vi "Find Labelled Disable Structure.vi"(8 "error in (no error)":errorcluster, 10 "Label":string, 11 "VI in":refnum<vi>) -> (0 "error out":errorcluster, 1 "Found?":bool, 2 "DisableStructure Refnum":refnum<vi>)   [LabVIEW 2018]
uses:
  <vilib>/Utility/traverseref.llb/TRef TravTarget.ctl
  <vilib>/Utility/error.llb/Error Cluster From Error Code.vi
  <vilib>/ErrorRing/Error Ring.xnode
  <vilib>/Utility/traverseref.llb/VI Scripting - Traverse.lvlib
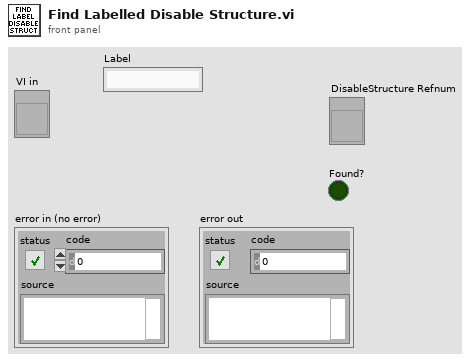
[diagram p1: front panel]
types:
  T1 = typedef "TRef TravTarget.ctl" = enum16{"FP", "BD", "Other"}
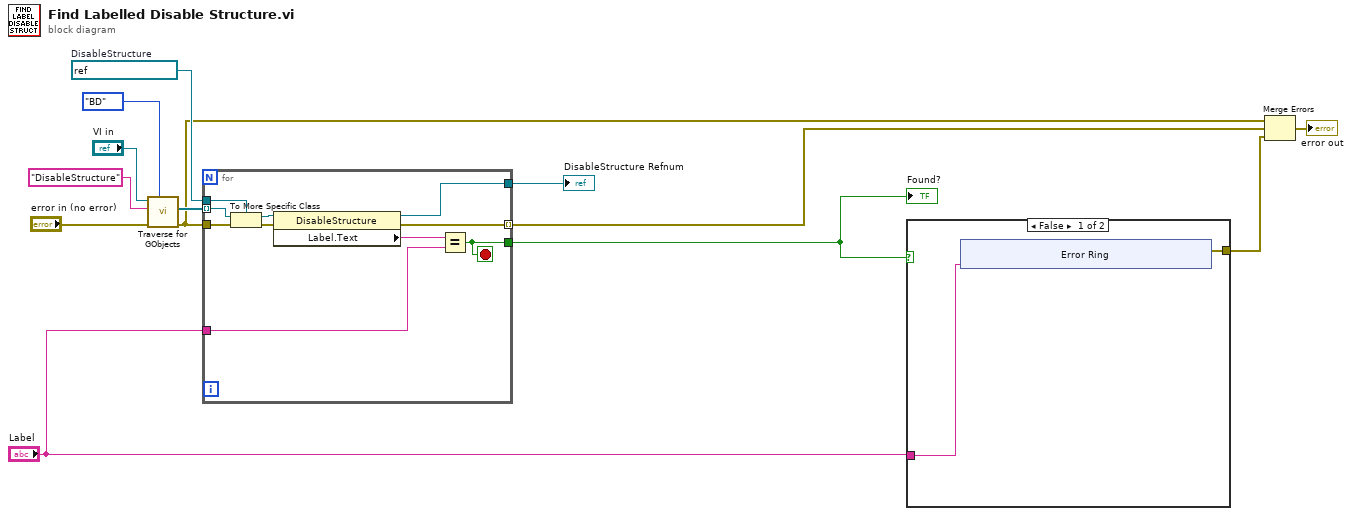
[diagram p0: block diagram]
diagram:
  w11 = refnum<vi> refnum  # DisableStructure
  n1 = call <vilib>:"Traverse for GObjects.vi"("Traverse Target"=TRef_TravTarget."BD", "error in (no error)"="error in (no error)", "Class Name"="DisableStructure", "VI Refnum"="VI in") -> ("error out"=w7:errorcluster, "References"=w8:refnum<vi>[])  [unwired: 4 in, 2 out]
  n2 = for {
    tunnel: w11 -> [w21]
    tunnel: w8 -> [w20] mode=indexing
    tunnel: "Label" -> [w16]
    tunnel: w7 -> [w23]
    tunnel: [w19] -> w6 mode=indexing
    tunnel: [w14] -> w1
    tunnel: [w15] -> w5
    stop <- w14 stop-if-true
    n3 = To More Specific Class(target class=w21, reference=w20, error in=w23) -> (specific class reference=w18:refnum<vi>, error out=w22:errorcluster)
    n4 = property class="DisableStructure"(reference=w18, error in=w22) -> (reference out=w15:refnum<vi>, error out=w19:errorcluster, "Label.Text"=w17:string)
    n5 = Equal?(x=w17, y=w16) -> (x = y?=w14:bool)
  }
  "Found?" <- w1
  "DisableStructure Refnum" <- w5
  n6 = case shown="False" w1 {
    tunnel: "Label" -> [w25 _]
    tunnel: [w24 _] -> w3
    frame False {
      n7 = xnode "Error Ring"("parameter 0"=w25) -> ("error out"=w24:errorcluster)
    }
    frame True {
    }
  }
  n8 = Merge Errors(w7, w6, w3) -> (→"error out":errorcluster)
